vi "ProbePlanAlign.vi"(3 "New Sensor":bool) -> (1 "Accept/Quit":bool)   [LabVIEW 2018]
uses:
  ProbePlanParams.vi
  InstrControl/ProbeStationControl/ProbeStationControl.lvclass
panel:
  in  "Old reference":bool
  in  "Already aligned":bool
  in  "align":bool
  out "Y1 2":i32
  out "X1 2":i32
  in  "Read probeplan reference":bool
  out "Y1280":i32
  out "X1280":i32
  in  "Readtop fiducial":bool
  out "Y1":i32
  out "X1":i32
  in  "Quit":bool
  in  "Accept":bool
  in  "Read bottom fiducial":bool
  # "Map Sensor to ProbePlan"
  # "X"
  # "Y"
  # "First Step:Align the sensor"
  # "as reference for bottom fiducial"
  # "as reference for top fiducial"
  # "Second step: locate the probeplan reference point on the sensor"
  # "as reference for ProbePlan"
  # "X:"
  # "Y:"
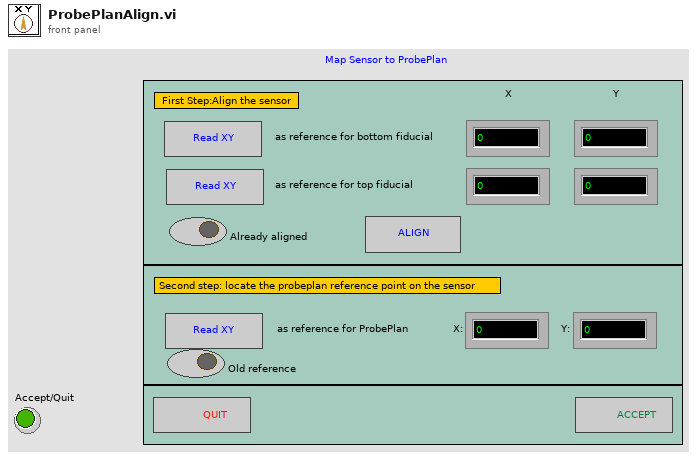
[diagram p1: front panel]
types:
  T1 = cluster{"Strip Number OUT":i32, "X0":i32, "Y0":i32, "X1":i32, "Y1":i32, "Xref":dbl, "Yref":dbl, "ProbePlan type":u32, "Inner pads offset":ext, "Outer pads offset":ext, "l_inner":ext, "l_outer":ext, "strip numbering":u16, "Device Orientation":ext, "Stagger offset":i32, "Yoffset":dbl, "Strip pitch":dbl, "Fiducail separation":dbl, "Radius":ext, "Relative strip angles":dbl, "Probeplan description":string, "ProbePlan array":cluster{"Region":string, "ProbePoints":cluster{"X":dbl, "Y":dbl, "Label":string, "CardViable?":bool}[]}[], "Test ProbePoints":cluster{"Regions Enabled":bool[], "From index":u32[], "To index":u32[]}}
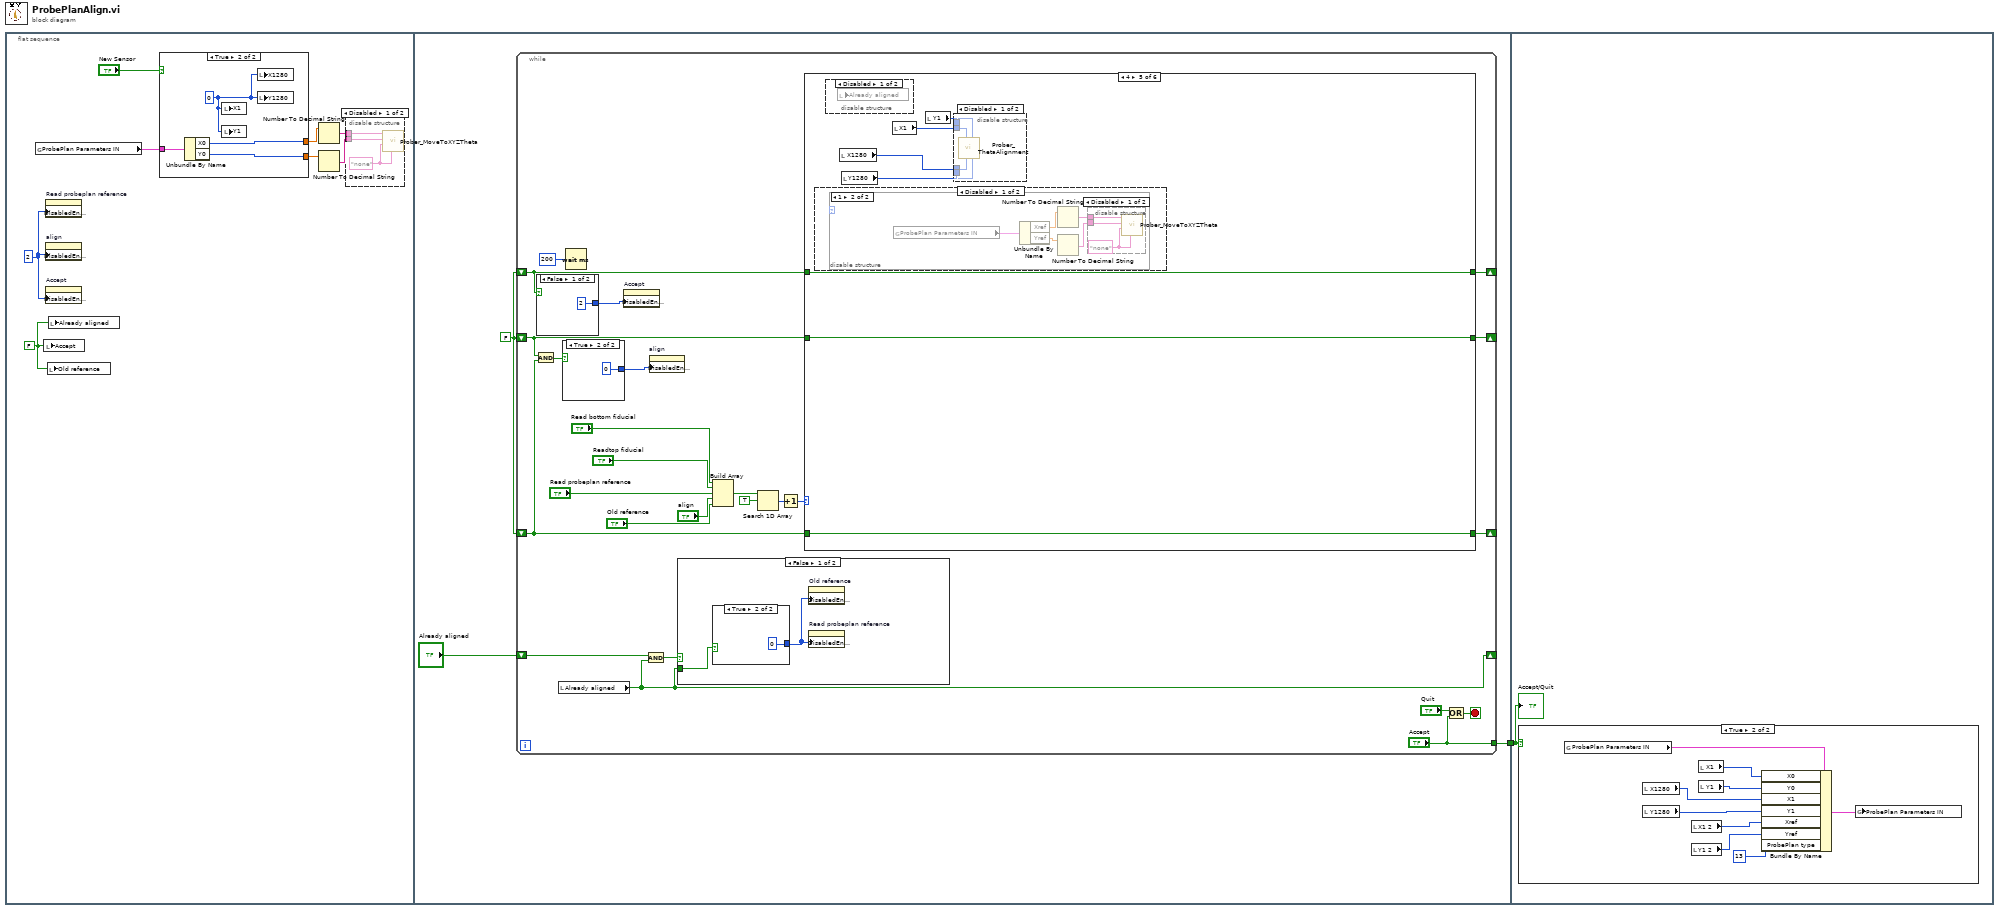
[diagram p0: block diagram]
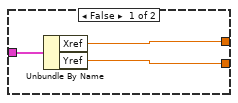
[diagram p3: hidden frame]
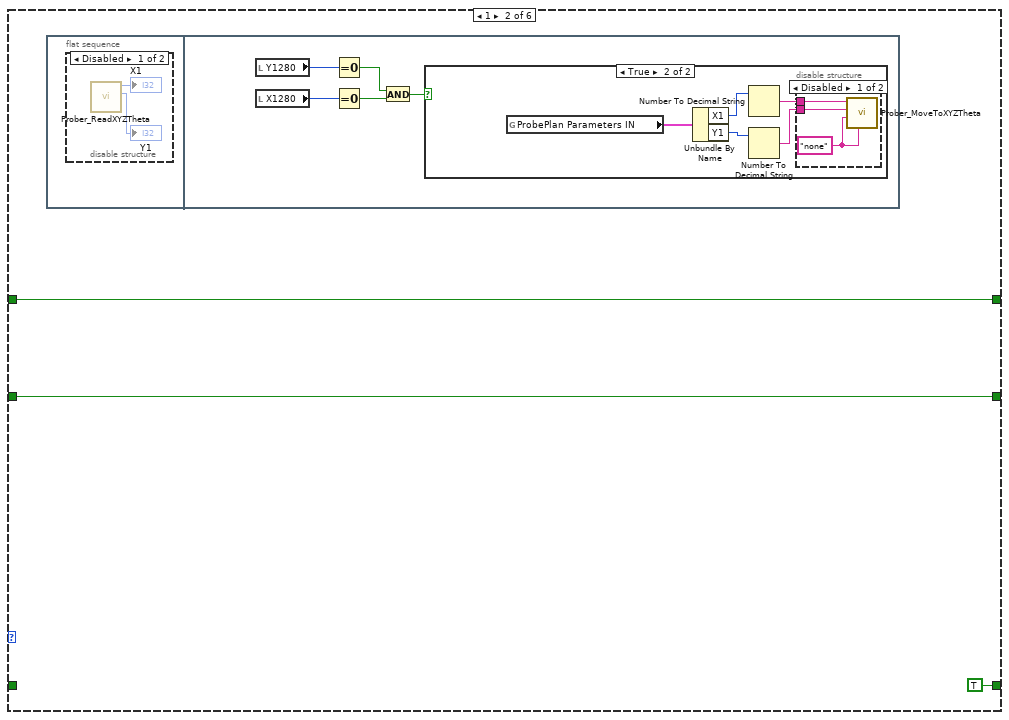
[diagram p5: hidden frame]
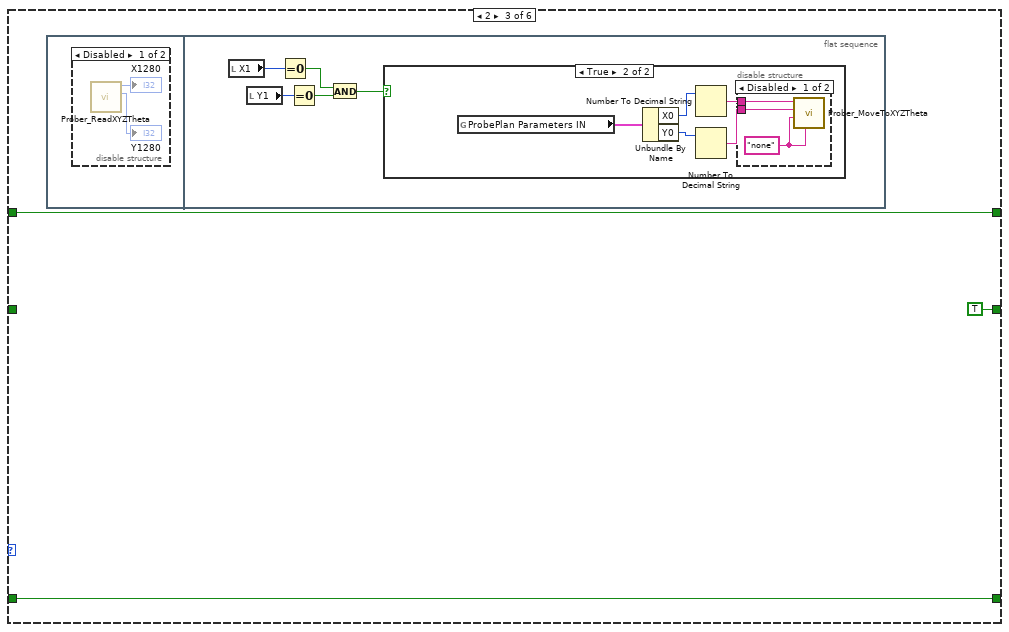
[diagram p9: hidden frame]
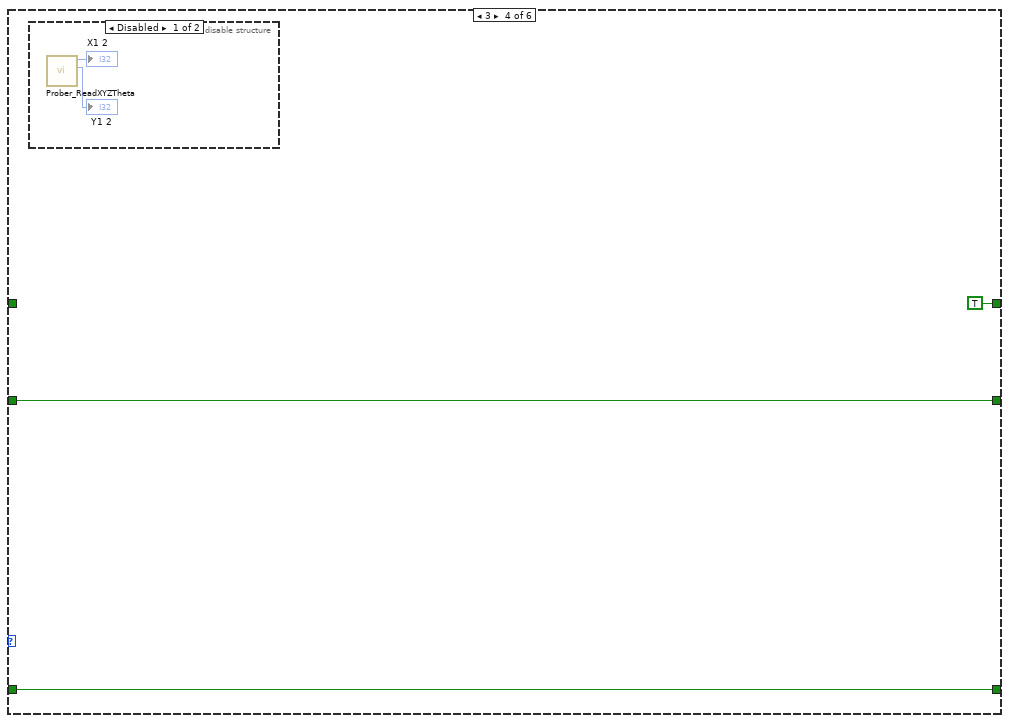
[diagram p13: hidden frame]
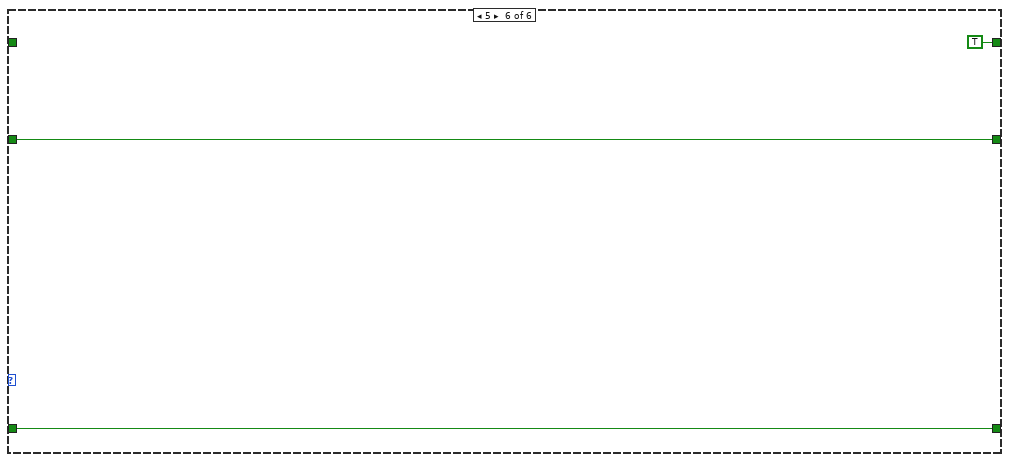
[diagram p20: hidden frame]
diagram:
  n1 = flat-sequence {
    tunnel: [w21] -> w1
    tunnel: w1 -> [w122]
    frame #0 {
      w9 = 2
      w8 = FALSE
      n2 = global read "ProbePlanParams.vi" "ProbePlan Parameters IN"() -> (w4:T1)
      n3 = local write "Accept"(w8) -> ()
      n4 = property on="Read probeplan reference" class="Bool"("DisabledEnum"=w9) -> ()  [unwired: 2 in, 2 out]
      n5 = property on="align" class="Bool"("DisabledEnum"=w9) -> ()  [unwired: 2 in, 2 out]
      n6 = property on="Accept" class="Bool (strict)"("DisabledEnum"=w9) -> ()  [unwired: 2 in, 2 out]
      n7 = local write "Old reference"(w8) -> ()
      n8 = local write "Already aligned"(w8) -> ()
      n9 = case shown="True" "New Sensor" {
        tunnel: w4 -> [w15 w19]
        tunnel: [w14 w18] -> w3
        tunnel: [w13 w17] -> w2
        frame False {
          n10 = Unbundle By Name(w15) -> ("Xref"=w14:dbl, "Yref"=w13:dbl)
        }
        frame True {
          w16 = 0
          n11 = Unbundle By Name(w19) -> ("X0"=w18:i32, "Y0"=w17:i32)
          n12 = local write "X1"(w16) -> ()
          n13 = local write "Y1"(w16) -> ()
          n14 = local write "X1280"(w16) -> ()
          n15 = local write "Y1280"(w16) -> ()
        }
      }
      n16 = Number To Decimal String(number=w3) -> (decimal integer string=w7:string)  [unwired: 1 in]
      n17 = Number To Decimal String(number=w2) -> (decimal integer string=w6:string)  [unwired: 1 in]
      n18 = disable-structure shown="Disabled" {
        disable-tunnel: w7 -> [w11 _]
        disable-tunnel: w6 -> [w10 _]
        frame Disabled {
          w12 = "none"
          n19 = call-dynamic "Prober_MoveToXYZTheta.vi"("Theta location [mdeg]"=w12, "Z location [µm]"=w12, "Y location [µm]"=w10, "X location [µm]"=w11) -> ()  [unwired: 5 in, 3 out]
        }
        frame Enabled {
        }
      }
    }
    frame #1 {
      w20 = FALSE
      n20 = while {
        shift-right: [w46] -> _
        shift-left: "Already aligned" -> [w29]
        tunnel: ["Accept"] -> w21
        shift-right: [w28] -> _
        shift-left: w20 -> [w31]
        shift-right: [w25] -> _
        shift-left: w20 -> [w26]
        shift-right: [w27] -> _
        shift-left: w20 -> [w30]
        stop <- w44 stop-if-true
        n21 = And(x=w31, y=w30) -> (x .and. y?=w33:bool)
        n22 = case shown="False" w26 {
          tunnel: [2 0] -> w35
          frame False {
          }
          frame True {
          }
        }
        n23 = local read "Already aligned"() -> (w46:bool)
        n24 = case shown="True" w33 {
          tunnel: [2 0] -> w34
          frame False {
          }
          frame True {
          }
        }
        n25 = Wait (ms)(milliseconds to wait=u32 200) -> ()  [unwired: 1 out]
        n26 = property on="Accept" class="Bool (strict)"("DisabledEnum"=w35) -> ()  [unwired: 2 in, 2 out]
        n27 = And(x=w29, y=w46) -> (x .and. y?=w47:bool)
        n28 = property on="align" class="Bool"("DisabledEnum"=w34) -> ()  [unwired: 2 in, 2 out]
        n29 = case shown="False" w47 {
          tunnel: w46 -> [w119 _]
          frame False {
            n30 = case shown="True" w119 {
              tunnel: [2 0] -> w118
              frame False {
              }
              frame True {
              }
            }
            n31 = property on="Old reference" class="Bool (strict)"("DisabledEnum"=w118) -> ()  [unwired: 2 in, 2 out]
            n32 = property on="Read probeplan reference" class="Bool"("DisabledEnum"=w118) -> ()  [unwired: 2 in, 2 out]
          }
          frame True {
          }
        }
        n33 = Build Array("Read bottom fiducial", "Readtop fiducial", "Read probeplan reference", "align", "Old reference") -> (w37:bool[])
        n34 = Search 1D Array(1D array=w37, element=TRUE) -> (index of element=w36:i32)  [unwired: 1 in]
        n35 = Increment(x=w36) -> (x+1=w32:i32)
        n36 = case shown="4" w32 {
          tunnel: w31 -> [w49 w51 _ w88 w93 w112]
          tunnel: w30 -> [w48 _ w71 w87 w94 w111]
          tunnel: [w49 w51 TRUE w88 w93 w112] -> w28
          tunnel: [w48 TRUE w71 w87 w94 w111] -> w27
          tunnel: w26 -> [w50 w53 w69 _ w92 _]
          tunnel: [w50 w53 w69 TRUE w92 TRUE] -> w25
          frame 0, Default {
          }
          frame 1 {
            n37 = flat-sequence {
              frame #0 {
                n38 = disable-structure shown="Disabled" {
                  frame Disabled {
                    n39 = call-dynamic "Prober_ReadXYZTheta.vi"() -> ("Y location [µm]"=→"Y1":i32, "X location [µm]"=→"X1":i32)  [unwired: 6 in, 4 out]
                  }
                  frame Enabled {
                  }
                }
              }
              frame #1 {
                n40 = local read "Y1280"() -> (w59:i32)
                n41 = local read "X1280"() -> (w60:i32)
                n42 = Equal To 0?(x=w59) -> (x = 0?=w58:bool)
                n43 = Equal To 0?(x=w60) -> (x = 0?=w57:bool)
                n44 = And(x=w58, y=w57) -> (x .and. y?=w56:bool)
                n45 = case shown="True" w56 {
                  frame False {
                  }
                  frame True {
                    n46 = global read "ProbePlanParams.vi" "ProbePlan Parameters IN"() -> (w63:T1)
                    n47 = Unbundle By Name(w63) -> ("X1"=w64:i32, "Y1"=w65:i32)
                    n48 = Number To Decimal String(number=w64) -> (decimal integer string=w61:string)  [unwired: 1 in]
                    n49 = Number To Decimal String(number=w65) -> (decimal integer string=w62:string)  [unwired: 1 in]
                    n50 = disable-structure shown="Disabled" {
                      disable-tunnel: w62 -> [w68 _]
                      disable-tunnel: w61 -> [w67 _]
                      frame Disabled {
                        w66 = "none"
                        n51 = call-dynamic "Prober_MoveToXYZTheta.vi"("Theta location [mdeg]"=w66, "Z location [µm]"=w66, "Y location [µm]"=w68, "X location [µm]"=w67) -> ()  [unwired: 5 in, 3 out]
                      }
                      frame Enabled {
                      }
                    }
                  }
                }
              }
            }
          }
          frame 2 {
            n52 = flat-sequence {
              frame #0 {
                n53 = disable-structure shown="Disabled" {
                  frame Disabled {
                    n54 = call-dynamic "Prober_ReadXYZTheta.vi"() -> ("Y location [µm]"=→"Y1280":i32, "X location [µm]"=→"X1280":i32)  [unwired: 6 in, 4 out]
                  }
                  frame Enabled {
                  }
                }
              }
              frame #1 {
                n55 = local read "X1"() -> (w78:i32)
                n56 = local read "Y1"() -> (w77:i32)
                n57 = Equal To 0?(x=w78) -> (x = 0?=w75:bool)
                n58 = Equal To 0?(x=w77) -> (x = 0?=w76:bool)
                n59 = And(x=w75, y=w76) -> (x .and. y?=w74:bool)
                n60 = case shown="True" w74 {
                  frame False {
                  }
                  frame True {
                    n61 = global read "ProbePlanParams.vi" "ProbePlan Parameters IN"() -> (w81:T1)
                    n62 = Unbundle By Name(w81) -> ("X0"=w82:i32, "Y0"=w83:i32)
                    n63 = Number To Decimal String(number=w82) -> (decimal integer string=w79:string)  [unwired: 1 in]
                    n64 = Number To Decimal String(number=w83) -> (decimal integer string=w80:string)  [unwired: 1 in]
                    n65 = disable-structure shown="Disabled" {
                      disable-tunnel: w80 -> [w86 _]
                      disable-tunnel: w79 -> [w85 _]
                      frame Disabled {
                        w84 = "none"
                        n66 = call-dynamic "Prober_MoveToXYZTheta.vi"("Theta location [mdeg]"=w84, "Z location [µm]"=w84, "Y location [µm]"=w86, "X location [µm]"=w85) -> ()  [unwired: 5 in, 3 out]
                      }
                      frame Enabled {
                      }
                    }
                  }
                }
              }
            }
          }
          frame 3 {
            n67 = disable-structure shown="Disabled" {
              frame Disabled {
                n68 = call-dynamic "Prober_ReadXYZTheta.vi"() -> ("Y location [µm]"=→"Y1 2":i32, "X location [µm]"=→"X1 2":i32)  [unwired: 6 in, 4 out]
              }
              frame Enabled {
              }
            }
          }
          frame 4 {
            n69 = disable-structure shown="Disabled" {
              frame Disabled {
                n70 = case shown="1" {
                  selector: _ -> [_ _]
                  frame 0, Default {
                  }
                  frame 1 {
                    n71 = global read "ProbePlanParams.vi" "ProbePlan Parameters IN"() -> (w101:T1)
                    n72 = Unbundle By Name(w101) -> ("Xref"=w102:dbl, "Yref"=w103:dbl)
                    n73 = Number To Decimal String(number=w102) -> (decimal integer string=w99:string)  [unwired: 1 in]
                    n74 = Number To Decimal String(number=w103) -> (decimal integer string=w100:string)  [unwired: 1 in]
                    n75 = disable-structure shown="Disabled" {
                      disable-tunnel: w100 -> [w106 _]
                      disable-tunnel: w99 -> [w105 _]
                      frame Disabled {
                        w104 = "none"
                        n76 = call-dynamic "Prober_MoveToXYZTheta.vi"("Theta location [mdeg]"=w104, "Z location [µm]"=w104, "Y location [µm]"=w106, "X location [µm]"=w105) -> ()  [unwired: 5 in, 3 out]
                      }
                      frame Enabled {
                      }
                    }
                  }
                }
              }
              frame Enabled {
              }
            }
            n77 = disable-structure shown="Disabled" {
              frame Disabled {
                n78 = local read "Already aligned"() -> ()  [unwired: 1 in]
              }
              frame Enabled {
              }
            }
            n79 = local read "X1280"() -> (w98:i32)
            n80 = local read "Y1280"() -> (w95:i32)
            n81 = local read "X1"() -> (w97:i32)
            n82 = local read "Y1"() -> (w96:i32)
            n83 = disable-structure shown="Disabled" {
              disable-tunnel: w98 -> [w110 _]
              disable-tunnel: w97 -> [w109 _]
              disable-tunnel: w96 -> [w108 _]
              disable-tunnel: w95 -> [w107 _]
              frame Disabled {
                n84 = call-dynamic "Prober_ThetaAlignment.vi"("y2"=w107, "y1"=w108, "x2"=w110, "x1"=w109) -> ()  [unwired: 4 in, 4 out]
              }
              frame Enabled {
              }
            }
          }
          frame 5 {
          }
        }
        n85 = Or(x="Quit", y="Accept") -> (x .or. y?=w44:bool)
      }
    }
    frame #2 {
      n86 = case shown="True" w122 {
        frame False {
        }
        frame True {
          n87 = global read "ProbePlanParams.vi" "ProbePlan Parameters IN"() -> (w127:T1)
          n88 = local read "X1280"() -> (w124:i32)
          n89 = local read "Y1280"() -> (w123:i32)
          n90 = local read "X1 2"() -> (w130:i32)
          n91 = local read "Y1 2"() -> (w129:i32)
          n92 = local read "X1"() -> (w126:i32)
          n93 = local read "Y1"() -> (w125:i32)
          n94 = Bundle By Name(cluster=w127, "X0"=w126, "Y0"=w125, "X1"=w124, "Y1"=w123, "Xref"=w130, "Yref"=w129, "ProbePlan type"=13) -> (w131:T1)
          n95 = global write "ProbePlanParams.vi" "ProbePlan Parameters IN"(w131) -> ()
        }
      }
      "Accept/Quit" <- w122
    }
  }
